vi "createReport.vi"(6 "date":string, 7 "obrn":string, 8 "error in (no error)":errorcluster, 9 "pruefer":string, 10 "Baugruppenname":string, 11 "DOM Document":refnum<k20>) -> (0 "error out":errorcluster, 2 "Report ref":refnum<k20>, 3 "dup DOM Document":refnum<k20>)   [LabVIEW 2013]
uses:
  <resource>/objmgr/DOMUserDefRef.rc
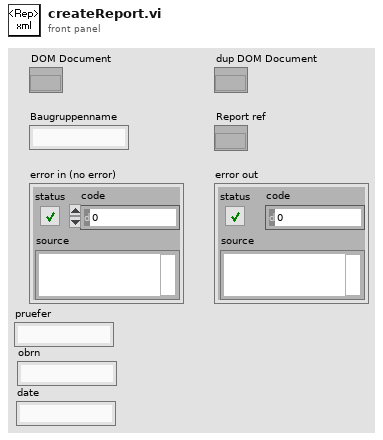
[diagram p1: front panel]
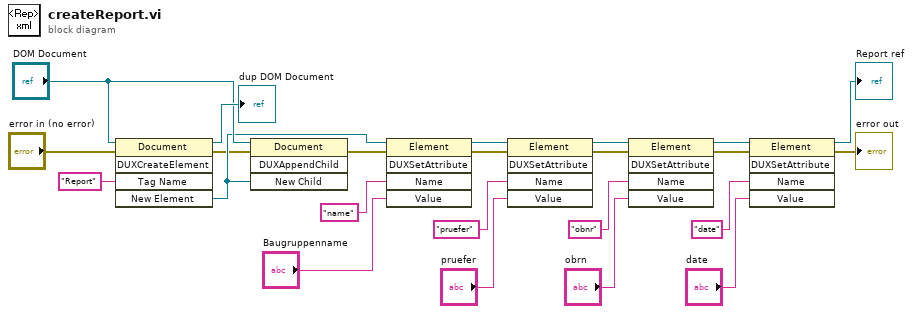
[diagram p0: block diagram]
diagram:
  n1 = invoke class="Document" method="DUXCreateElement"(reference="DOM Document", error in="error in (no error)", "Tag Name"="Report" ("Qualified Name")) -> (reference out=→"dup DOM Document":refnum<k20>, error out=w8:errorcluster, "New Element"=w9:refnum<k20>)  [unwired: 2 in, 2 out]
  n2 = invoke class="Document" method="DUXAppendChild"(reference="DOM Document", error in=w8, "New Child"=w9) -> (error out=w7:errorcluster)  [unwired: 1 in, 3 out]
  n3 = invoke class="Element" method="DUXSetAttribute"(reference=w9, error in=w7, "Name"="name" ("Report Name"), "Value"="Baugruppenname") -> (reference out=w18:refnum<k20>, error out=w17:errorcluster)  [unwired: 1 in, 3 out]
  n4 = invoke class="Element" method="DUXSetAttribute"(reference=w18, error in=w17, "Name"="pruefer", "Value"="pruefer") -> (reference out=w16:refnum<k20>, error out=w15:errorcluster)  [unwired: 1 in, 3 out]
  n5 = invoke class="Element" method="DUXSetAttribute"(reference=w16, error in=w15, "Name"="obnr", "Value"="obrn") -> (reference out=w6:refnum<k20>, error out=w5:errorcluster)  [unwired: 1 in, 3 out]
  n6 = invoke class="Element" method="DUXSetAttribute"(reference=w6, error in=w5, "Name"="date", "Value"="date") -> (reference out=→"Report ref":refnum<k20>, error out=→"error out":errorcluster)  [unwired: 1 in, 3 out]
